vi "TCL Get Message.vi"() -> (0 "Text":string, 1 "TCL Message Type":T1(ring)=enum."Address=")   [LabVIEW 2019]
panel:
  in  "Timeout ms (-1)":i32=-1
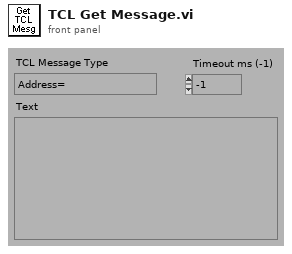
[diagram p1: front panel]
types:
  T1 = enum16{"No Message", "Bad Message", "NewEventFile", "NewBaseFile", "Event=", "Ping=", "Address=", "Stop"}
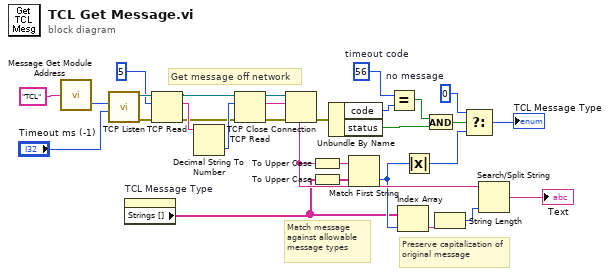
[diagram p0: block diagram]
diagram:
  w10 = 0  # no message
  w13 = 56  # timeout code
  # "Get message off network"
  # "Match message against allowable message types"
  # "Preserve capitalization of original message"
  n1 = call "Message Get Module Address.vi"("Module"="TCL") -> ("Port"=w7:u16)  [unwired: 1 out]
  n2 = call <vilib>:"TCP Listen.vi"("timeout ms (wait forever: -1)"="Timeout ms (-1)", "port"=w7) -> ("error out"=w24:errorcluster, "connection ID"=w25:refnum<k5>)  [unwired: 5 in, 3 out]
  n3 = property on="TCL Message Type" class="Enum (strict)"() -> ("Strings []"=w6:string[])  [unwired: 2 in, 2 out]
  n4 = TCP Read(connection ID=w25, bytes to read=5 ("size of message length"), error in (no error)=w24) -> (connection ID out=w20:refnum<k5>, data out=w22:string, error out=w19:errorcluster)  [unwired: 2 in]
  n5 = Decimal String To Number(string=w22) -> (number=w21:i32)  [unwired: 2 in, 1 out]
  n6 = TCP Read(connection ID=w20, bytes to read=w21, error in (no error)=w19) -> (connection ID out=w1:refnum<k5>, data out=w18:string, error out=w3:errorcluster)  [unwired: 2 in]
  n7 = TCP Close Connection(connection ID=w1, error in (no error)=w3) -> (error out=w2:errorcluster)  [unwired: 1 in, 1 out]
  n8 = To Upper Case(1:w18) -> (0:w29:string)
  n9 = To Upper Case(1:w6) -> (0:w28:string[])
  n10 = Unbundle By Name(w2) -> ("code"=w14:i32, "status"=w16:bool)
  n11 = Match First String(2:w28, 3:w29) -> (0:w12:i32)  [unwired: 1 out]
  n12 = Equal?(x=w13, y=w14) -> (x = y?=w15:bool)
  n13 = Index Array(array=w6, index=w12) -> (element=w26:string)
  n14 = Absolute Value(x=w12) -> (abs(x)=w9:i32)
  n15 = And(x=w15, y=w16) -> (x .and. y?=w11:bool)
  n16 = String Length(string=w26) -> (length=w27:i32)
  n17 = Select(t=w10, s=w11, f=w9) -> (s? t:f=→"TCL Message Type":i32)
  n18 = Search/Split String(string=w18, offset (0)=w27) -> (match + rest of string=→"Text":string)  [unwired: 1 in, 2 out]
